vi "Playbook_v2_Init.vi"(0 "object in":refnum<class "Playbook_v2.lvclass">, 5 "error in (no error)":errorcluster) -> (14 "object out":refnum<class "Playbook_v2.lvclass">, 19 "error out":errorcluster)   [LabVIEW 2023, in "Playbook_v2.lvclass"]
uses:
  Playbook_v2.lvclass
  NewPlays/StandardAttackPlay_class/StandardAttackPlay.lvclass
  C:/Users/ebert/Documents/codes/SSL/repo/SSL_AI/NewSTP/NewPlays/Play_v2_class/Play_v2.lvclass
  STP_Parameters/OffensivePlays_v2.ctl
  Playbook_v2.lvclass/Playbook_v2.ctl
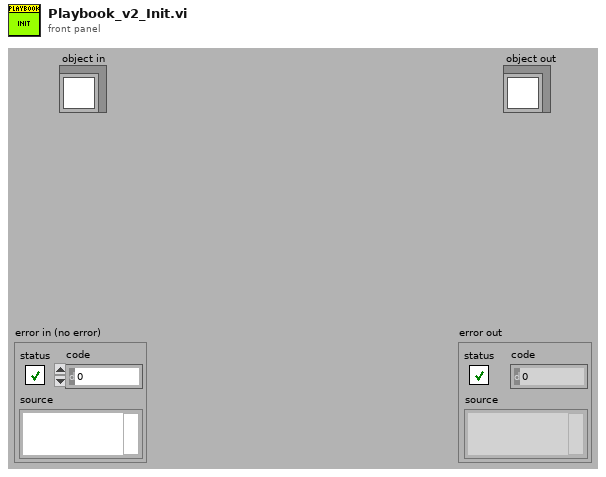
[diagram p1: front panel]
types:
  T1 = typedef "OffensivePlays_v2.ctl" = enum16{"StandardAttack"}
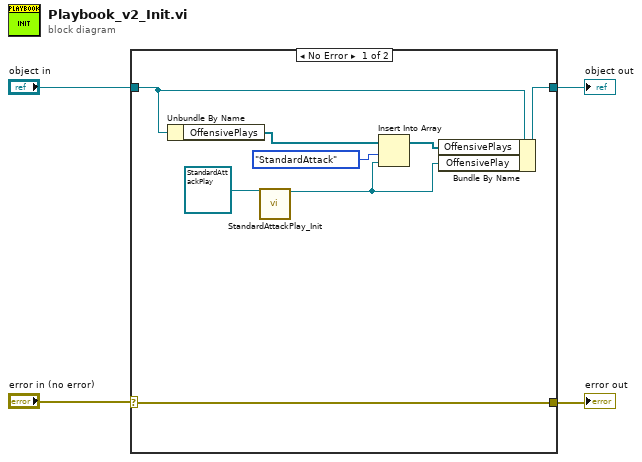
[diagram p0: block diagram]
diagram:
  n1 = case shown="No Error" "error in (no error)" {
    selector: "error in (no error)" -> [w11 w13]
    tunnel: "object in" -> [w7 w14]
    tunnel: [w12 w14] -> w3
    tunnel: [w11 w13] -> w1
    frame No Error {
      n2 = Unbundle By Name(w7) -> ("OffensivePlays"=w6:refnum<class "Play_v2.lvclass">[])
      n3 = call "StandardAttackPlay_Init.vi"("object in"=refnum<class "StandardAttackPlay.lvclass"> refnum ("StandardAttackPlay")) -> ("object out"=w8:refnum<class "StandardAttackPlay.lvclass">)  [unwired: 17 in, 1 out]
      n4 = Insert Into Array(array=w6, index=OffensivePlays_v2."StandardAttack" ("Enum"), new element=w8) -> (w5:refnum<class "Play_v2.lvclass">[])
      n5 = Bundle By Name(cluster=w7, "OffensivePlays"=w5, "OffensivePlay"=w8) -> (w12:refnum<class "Playbook_v2.lvclass">)
    }
    frame Error {
    }
  }
  "object out" <- w3
  "error out" <- w1
